vi "Write Base I32.vi"(5 "timestamps":timestamp[](array[numeric]), 7 "index_channel":u32, 8 "error in":errorcluster, 9 "data":i32[][](array[numeric]), 10 "channels":u32[](array[numeric]), 11 "Writer":refnum<class "Synnax Writer.lvclass">) -> (0 "error out":errorcluster, 3 "Writer Out":refnum<class "Synnax Writer.lvclass">)   [LabVIEW 2026, in "synnax_clib.lvlib" / "Synnax Writer.lvclass"]
doc: "SYNNAX_EXPORT int32_t synnax_writer_write(\n SynnaxWriter writer,\n uint32_t channel,\n const double *data,\n uint64_t sample_count,\n SynnaxError err\n);"
uses:
  Synnax Writer.lvclass
  Synnax Writer.lvclass/Synnax Writer.ctl
  synnax_clib.lvlib
  synnax_clib.dll
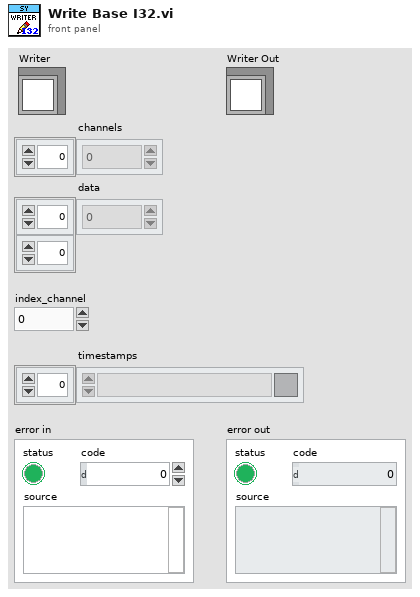
[diagram p1: front panel]
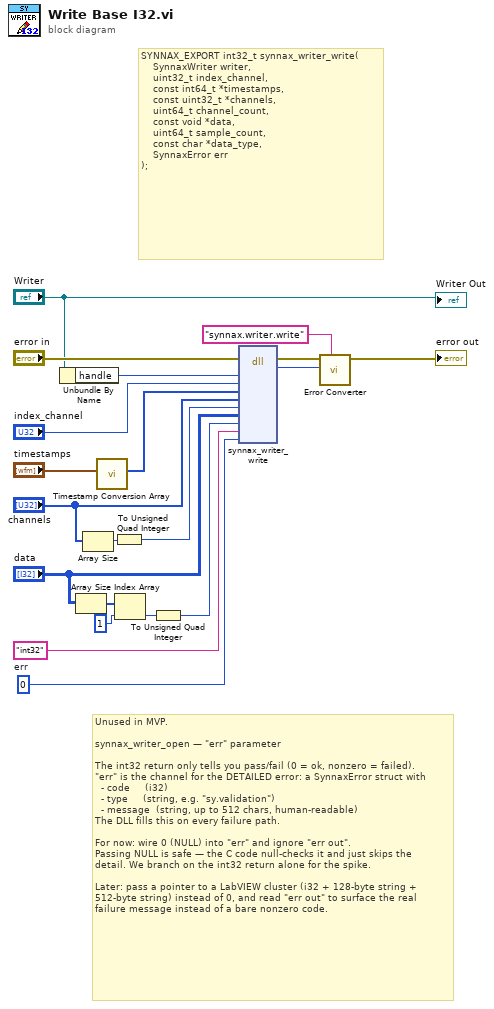
[diagram p0: block diagram]
diagram:
  w19 = u64 0  # err
  # "Unused in MVP.\n\nsynnax_writer_open — \"err\" parameter\n\nThe int32 return only tells you pass/fail (0 = ok, nonzero = failed).\n\"err\" is the channel for the DETAILED error: a SynnaxError struct with\n  - code     (i32)\n  - type     (string, e.g. \"sy.validation\")\n  - message  (string, up to 512 chars, human-readable)\nThe DLL fills this on every failure path.\n\nFor now: wire 0 (NULL) into \"err\" and ignore \"err out\".\nPassing NULL is safe — the C code null-checks it and just skips the\ndetail. We branch on the int32 return alone for the spike.\n\nLater: pass a pointer to a LabVIEW cluster (i32 + 128-byte string +\n512-byte string) instead of 0, and read \"err out\" to surface the real\nfailure message instead of a bare nonzero code."
  # "SYNNAX_EXPORT int32_t synnax_writer_write(\n    SynnaxWriter writer,\n    uint32_t index_channel,\n    const int64_t *timestamps,\n    const uint32_t *channels,\n    uint64_t channel_count,\n    const void *data,\n    uint64_t sample_count,\n    const char *data_type,\n    SynnaxError err\n);"
  n1 = Unbundle By Name("Writer") -> ("handle"=w2:u64)
  n2 = Array Size(array="data") -> (size(s)=w7:i32[])
  n3 = Array Size(array="channels") -> (size(s)=w13:i32)
  n4 = call "Timestamp Conversion Array.vi"("timestamps"="timestamps") -> ("timestamps (ns)"=w3:i64[])  [unwired: 9 in]
  n5 = To Unsigned Quad Integer(1:w13) -> (0:w12:u64)
  n6 = Index Array(array=w7, index=1) -> (element=w6:i32)
  n7 = To Unsigned Quad Integer(1:w6) -> (0:w9:u64)
  n8 = dll-call lib="C/synnax/client/labview/synnax_clib.*" fn="synnax_writer_write"(error in="error in", "writer"=w2, "index_channel"="index_channel", "timestamps"=w3, "channels"="channels", "channel_count"=w12, "data"="data", "sample_count"=w9, "data_type"="int32", "err"=w19) -> (error out=w18:errorcluster, "return type"=w17:i32)  [unwired: 11 in, 1 out]
  n9 = call "Error Converter.vi"("source"="synnax.writer.write", "error code"=w17, "error in (no error)"=w18) -> ("error out"=→"error out":errorcluster)  [unwired: 8 in]
  "Writer Out" <- "Writer"
